vi "KRH Arm PID (SubVI).vi"(4 "Actual Angle":dbl, 5 "Arm Control":T1, 6 "PID Settings":T3, 7 "PID Limits":cluster{"Upper Limit":dbl, "Lower Limit":dbl}) -> (0 "Arm Status":T2, 3 "output":dbl)   [LabVIEW 2015]
uses:
  <vilib>/addons/control/pid/pid.llb/PID (DBL).vi
  <vilib>/addons/control/pid/NI_PID_pid.lvlib
panel:
  out "Arm Angle Chart":dbl(graph)
  out "PID Output Chart":dbl(graph)
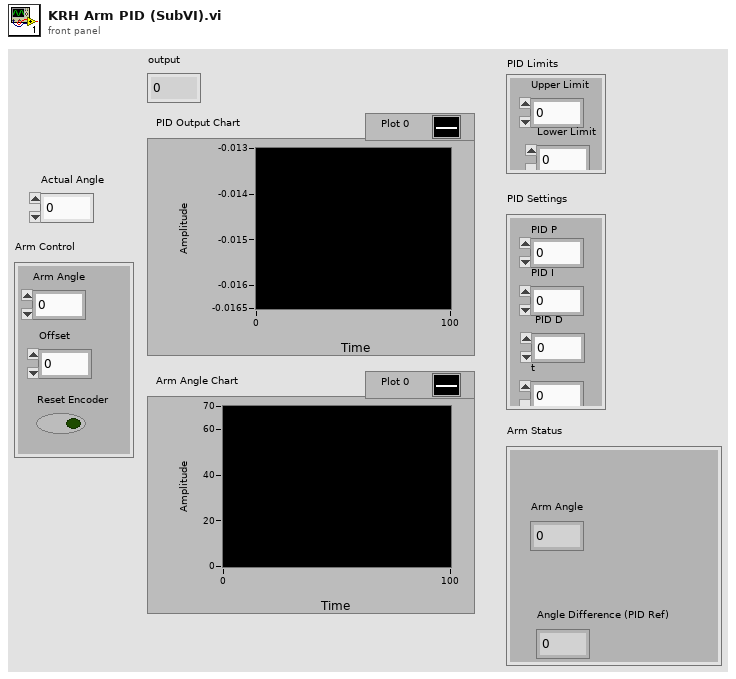
[diagram p1: front panel]
types:
  T1 = cluster{"Arm Angle":dbl, "Offset":dbl, "Reset Encoder":bool}
  T2 = cluster{"Arm Angle":dbl, "Angle Difference (PID Ref)":dbl}
  T3 = cluster{"PID P":dbl, "PID I":dbl, " PID D":dbl, "t":dbl}
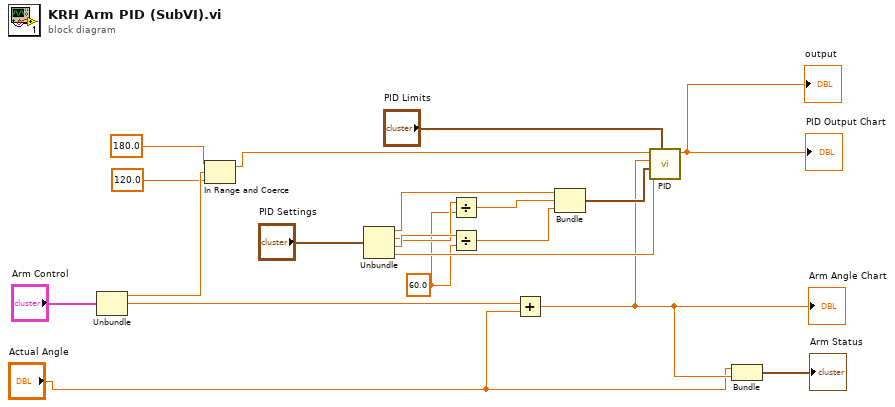
[diagram p0: block diagram]
diagram:
  w6 = 60.0
  n1 = Unbundle("Arm Control") -> ("Arm Angle"=w3:dbl, "Offset"=w12:dbl)  [unwired: 1 out]
  n2 = In Range and Coerce(upper limit=180.0, x=w3, lower limit=120.0) -> (coerced(x)=w4:dbl)  [unwired: 1 out]
  n3 = Unbundle("PID Settings") -> ("PID P"=w8:dbl, "PID I"=w10:dbl, "PID D"=w11:dbl, "t"=w17:dbl)
  n4 = Divide(x=w10, y=w6) -> (x/y=w7:dbl)
  n5 = Divide(x=w11, y=w6) -> (x/y=w9:dbl)
  n6 = Add(x=w12, y="Actual Angle") -> (x+y=w14:dbl)
  "Arm Angle Chart" <- w14
  n7 = Bundle("PID P"=w8, w7, w9) -> (w16:cluster{"PID P":dbl, dbl, dbl})  [unwired: 1 in]
  n8 = call-poly <vilib>:"PID.vi"("output range"="PID Limits", "dt (s)"=w17, "PID gains"=w16, "process variable"=w14, "setpoint"=w4) -> ("output"=→"PID Output Chart" →"output":dbl)  [unwired: 5 in, 1 out]
  n9 = Bundle("Actual Angle"="Actual Angle", w14) -> (→"Arm Status":cluster{"Actual Angle":dbl, dbl})  [unwired: 1 in]
